vi "Configure S-parameter Correction.vi"(8 "error in (no error)":errorcluster, 9 "S-parameter Table Name (\"DEFAULT\")":string="\"DEFAULT\"", 10 "Enable S-parameter Correction (T: Enable)":bool=TRUE, 11 "VISA resource name":refnum<visa-resource-name>) -> (0 "error out":errorcluster, 3 "VISA resource name out":refnum<visa-resource-name>)   [LabVIEW 2014, in "Agilent U2000 Series.lvlib"]
doc: "Enables or disables the S-parameter correction and select the S-parameter table to be used for S-parameter correction.\n\nNote:\nThis VI has been obsoleted from the driver and is included for compatibility with existing applications. \n New applications should use the new Public VIs Configure S-parameter Table and Enable S-parameter Table."
uses:
  Agilent U2000 Series.lvlib
panel:
  # "Note:\nThis VI has been obsoleted from the driver and is included for compatibility with existing applications. \n New applications should use the new Public VIs Configure S-parameter Table and Enable S-parameter Table."
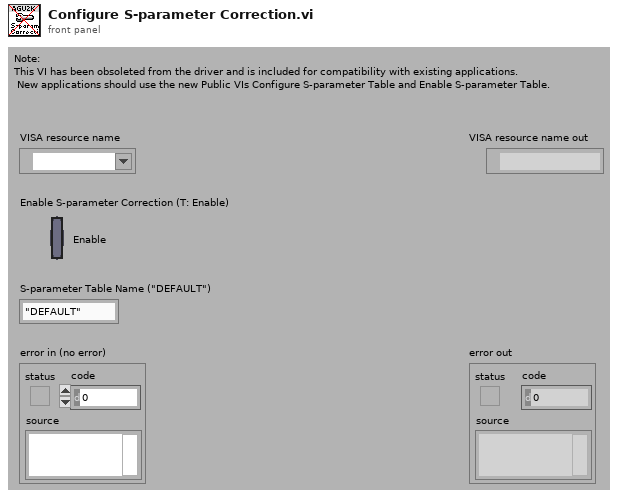
[diagram p1: front panel]
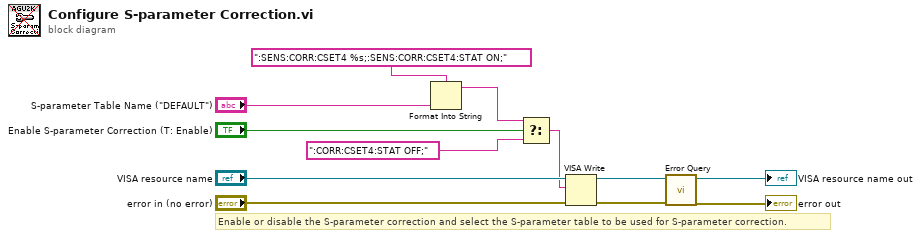
[diagram p0: block diagram]
diagram:
  # "Enable or disable the S-parameter correction and select the S-parameter table to be used for S-parameter correction."
  n1 = Format Into String(format string=":SENS:CORR:CSET4 %s;:SENS:CORR:CSET4:STAT ON;", "S-parameter Table Name (\"DEFAULT\")") -> (resulting string=w1:string)  [unwired: 2 in, 1 out]
  n2 = Select(t=w1, s="Enable S-parameter Correction (T: Enable)", f=":CORR:CSET4:STAT OFF;") -> (s? t:f=w3:string)
  n3 = VISA Write(VISA resource name="VISA resource name", write buffer=w3, error in (no error)="error in (no error)") -> (VISA resource name out=w8:refnum<visa-resource-name>, error out=w7:errorcluster)  [unwired: 1 out]
  n4 = call "Error Query.vi"("error in (no error)"=w7, "VISA resource name"=w8) -> ("error out"=→"error out":errorcluster, "VISA resource name out"=→"VISA resource name out":refnum<visa-resource-name>)  [unwired: 6 in, 2 out]
